vi "글로벌변수_2.vi"() -> ()   [LabVIEW 2013]
panel:
  out "웨이브폼 차트":dbl(graph)
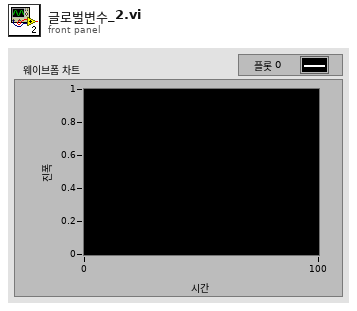
[diagram p1: front panel]
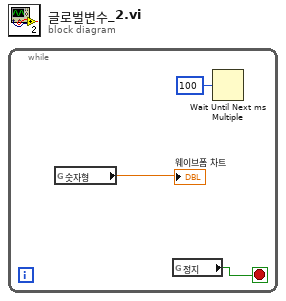
[diagram p0: block diagram]
diagram:
  n1 = while {
    stop <- w1 stop-if-true
    n2 = global read "글로벌_변수VI.vi" "숫자형"() -> (→"웨이브폼 차트":dbl)
    n3 = global read "글로벌_변수VI.vi" "정지"() -> (w1:bool)
    n4 = Wait Until Next ms Multiple(millisecond multiple=u32 100 ("ms 배수")) -> ()  [unwired: 1 out]
  }
